vi "VersionStrings.GetProjectPaths.vi"(1 "Version Build Info":T1={"VeriStand Version"="2013 SP1", "TestStand Version"="2013", "New VS Assembly Version"="2013.0.0.0", "New TS Assembly Version"="5.1.0.226", "VeriStand Steps Version String"="14.0.5.0", "Project Paths"={"MiscHelperVIs Project Path"="", "RTSequenceVIs Project Path"="", "Set Channels Project Path"="", "TS VS Logger Project Path"="", "VeriStand.exe Install Path"="", "NI_VeristandTypes.ini File Path"="", "Workspace Path"="", "VeristandSteps.csproj File Path"="", "Silent Veristand Project Path"=""}, "New TS Interop Assembly Version"="1.2.3.4", "New TS Utility Assembly Version"="5.6.7.8", "New VS Assembly Version (GAC)"="4.0.2016.0.9.9", "dotNET .config File Paths"={"MiscHelperVIs Project .config File Path"=path "C:/Users/Public/Documents/Git-Source/VeriStand-Custom-Steps-For-TestStand/Source/LabVIEW Code/Misc/MiscHelperVIs.lvproj.config", "RT Sequence VIs Project .config File Path"=path "C:/Users/Public/Documents/Git-Source/VeriStand-Custom-Steps-For-TestStand/Source/LabVIEW Code/RT Sequence/RTSequenceVIs.lvproj.config", "Set Channels Project .config File Path"=path "C:/Users/Public/Documents/Git-Source/VeriStand-Custom-Steps-For-TestStand/Source/LabVIEW Code/Set Channels/Set Channels.lvproj.config", "TS VS Logger Project .config File Path"=path "C:/Users/Public/Documents/Git-Source/VeriStand-Custom-Steps-For-TestStand/Source/LabVIEW Code/TS VS Logger/TS VS Logger.lvproj.config", "Silent Veristand Project .config File Path"=path "C:/Users/Public/Documents/Git-Source/VeriStand-Custom-Steps-For-TestStand/Source/LabVIEW Code/VeriStand Silent Start/SilentVS.lvproj.config"}}) -> (0 "Version Build Info out":T1={"VeriStand Version"="2013 SP1", "TestStand Version"="2013", "New VS Assembly Version"="2013.0.0.0", "New TS Assembly Version"="5.1.0.226", "VeriStand Steps Version String"="14.0.5.0", "Project Paths"={"MiscHelperVIs Project Path"="", "RTSequenceVIs Project Path"="", "Set Channels Project Path"="", "TS VS Logger Project Path"="", "VeriStand.exe Install Path"="", "NI_VeristandTypes.ini File Path"="", "Workspace Path"="", "VeristandSteps.csproj File Path"="", "Silent Veristand Project Path"=""}, "New TS Interop Assembly Version"="1.2.3.4", "New TS Utility Assembly Version"="5.6.7.8", "New VS Assembly Version (GAC)"="4.0.2016.0.9.9", "dotNET .config File Paths"={"MiscHelperVIs Project .config File Path"=path "C:/Users/Public/Documents/Git-Source/VeriStand-Custom-Steps-For-TestStand/Source/LabVIEW Code/Misc/MiscHelperVIs.lvproj.config", "RT Sequence VIs Project .config File Path"=path "C:/Users/Public/Documents/Git-Source/VeriStand-Custom-Steps-For-TestStand/Source/LabVIEW Code/RT Sequence/RTSequenceVIs.lvproj.config", "Set Channels Project .config File Path"=path "C:/Users/Public/Documents/Git-Source/VeriStand-Custom-Steps-For-TestStand/Source/LabVIEW Code/Set Channels/Set Channels.lvproj.config", "TS VS Logger Project .config File Path"=path "C:/Users/Public/Documents/Git-Source/VeriStand-Custom-Steps-For-TestStand/Source/LabVIEW Code/TS VS Logger/TS VS Logger.lvproj.config", "Silent Veristand Project .config File Path"=path "C:/Users/Public/Documents/Git-Source/VeriStand-Custom-Steps-For-TestStand/Source/LabVIEW Code/VeriStand Silent Start/SilentVS.lvproj.config"}})   [LabVIEW 2014, in "VeriStand Steps Version Mutation.lvlib"]
uses:
  VeriStand Steps Version Mutation.lvlib
  Types/Version Build Information.ctl
  Types/Project Paths Cluster.ctl
  Types/dotNET Config File Paths Cluster.ctl
  Types/Constants.vi
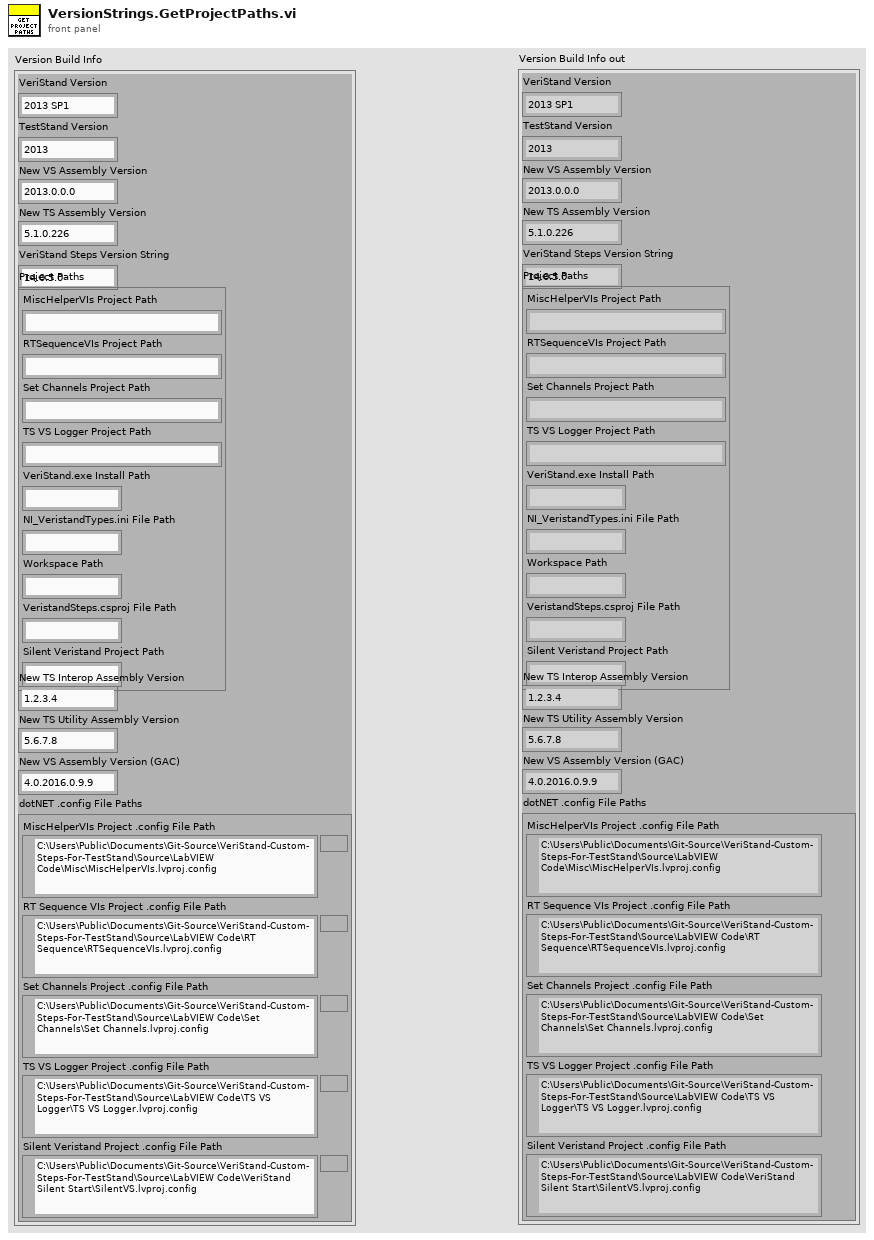
[diagram p1: front panel]
types:
  T1 = typedef "VeriStand Steps Version Mutation.lvlib/Version Build Information.ctl" = cluster{"VeriStand Version":string, "TestStand Version":string, "New VS Assembly Version":string, "New TS Assembly Version":string, "VeriStand Steps Version String":string, "Project Paths":T2, "New TS Interop Assembly Version":string, "New TS Utility Assembly Version":string, "New VS Assembly Version (GAC)":string, "dotNET .config File Paths":T3}
  T2 = typedef "VeriStand Steps Version Mutation.lvlib/Project Paths Cluster.ctl" = cluster{"MiscHelperVIs Project Path":string, "RTSequenceVIs Project Path":string, "Set Channels Project Path":string, "TS VS Logger Project Path":string, "VeriStand.exe Install Path":string, "NI_VeristandTypes.ini File Path":string, "Workspace Path":string, "VeristandSteps.csproj File Path":string, "Silent Veristand Project Path":string}
  T3 = typedef "VeriStand Steps Version Mutation.lvlib/dotNET Config File Paths Cluster.ctl" = cluster{"MiscHelperVIs Project .config File Path":path, "RT Sequence VIs Project .config File Path":path, "Set Channels Project .config File Path":path, "TS VS Logger Project .config File Path":path, "Silent Veristand Project .config File Path":path}
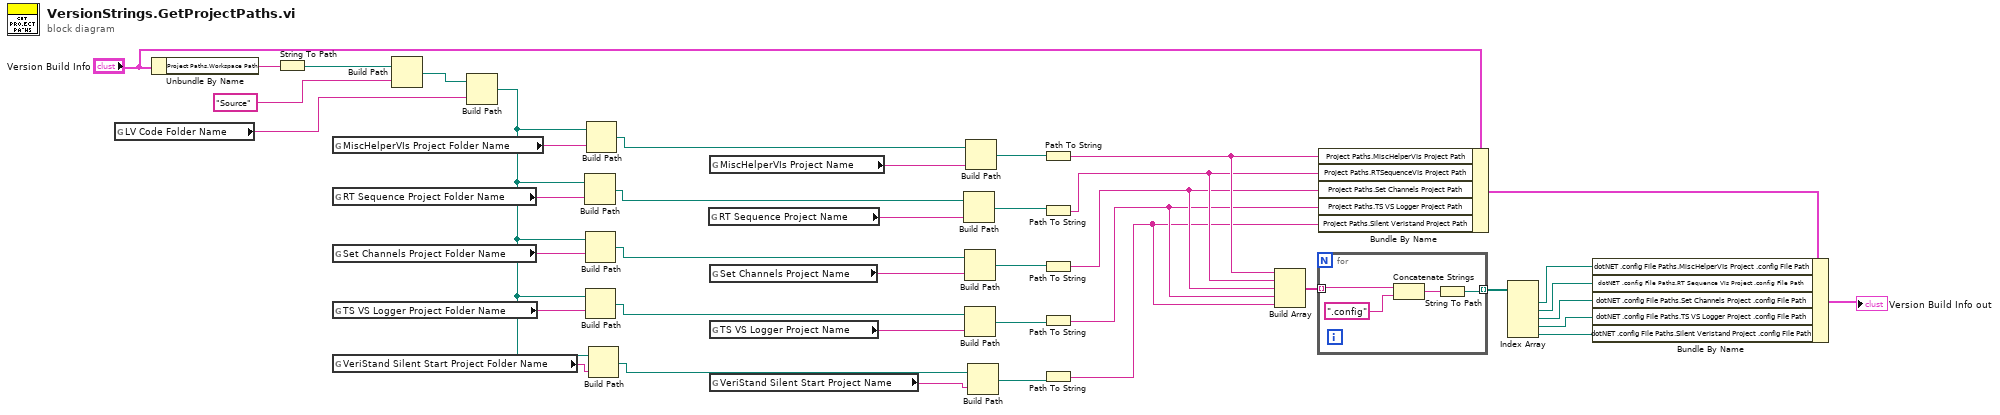
[diagram p0: block diagram]
diagram:
  n1 = global read "Constants.vi" "LV Code Folder Name"() -> (w38:string)
  n2 = Unbundle By Name("Version Build Info") -> ("Project Paths.Workspace Path"=w41:string)
  n3 = String To Path(string=w41) -> (path=w40:path)
  n4 = global read "Constants.vi" "MiscHelperVIs Project Folder Name"() -> (w37:string)
  n5 = global read "Constants.vi" "RT Sequence Project Folder Name"() -> (w35:string)
  n6 = global read "Constants.vi" "Set Channels Project Folder Name"() -> (w34:string)
  n7 = global read "Constants.vi" "TS VS Logger Project Folder Name"() -> (w33:string)
  n8 = global read "Constants.vi" "VeriStand Silent Start Project Folder Name"() -> (w31:string)
  n9 = Build Path(base path=w40, name or relative path="Source") -> (appended path=w36:path)
  n10 = Build Path(base path=w36, name or relative path=w38) -> (appended path=w32:path)
  n11 = Build Path(base path=w32, name or relative path=w35) -> (appended path=w29:path)
  n12 = Build Path(base path=w32, name or relative path=w34) -> (appended path=w28:path)
  n13 = Build Path(base path=w32, name or relative path=w33) -> (appended path=w27:path)
  n14 = Build Path(base path=w32, name or relative path=w37) -> (appended path=w30:path)
  n15 = Build Path(base path=w32, name or relative path=w31) -> (appended path=w26:path)
  n16 = global read "Constants.vi" "RT Sequence Project Name"() -> (w24:string)
  n17 = global read "Constants.vi" "MiscHelperVIs Project Name"() -> (w25:string)
  n18 = global read "Constants.vi" "Set Channels Project Name"() -> (w23:string)
  n19 = global read "Constants.vi" "TS VS Logger Project Name"() -> (w22:string)
  n20 = global read "Constants.vi" "VeriStand Silent Start Project Name"() -> (w21:string)
  n21 = Build Path(base path=w29, name or relative path=w24) -> (appended path=w18:path)
  n22 = Build Path(base path=w28, name or relative path=w23) -> (appended path=w17:path)
  n23 = Build Path(base path=w27, name or relative path=w22) -> (appended path=w16:path)
  n24 = Build Path(base path=w30, name or relative path=w25) -> (appended path=w19:path)
  n25 = Build Path(base path=w26, name or relative path=w21) -> (appended path=w15:path)
  n26 = Path To String(path=w19) -> (string=w14:string)
  n27 = Path To String(path=w18) -> (string=w13:string)
  n28 = Path To String(path=w17) -> (string=w12:string)
  n29 = Path To String(path=w16) -> (string=w11:string)
  n30 = Path To String(path=w15) -> (string=w10:string)
  n31 = Build Array(w14, w13, w12, w11, w10) -> (w9:string[])
  n32 = for {
    tunnel: w9 -> [w45] mode=indexing
    tunnel: [w42] -> w7 mode=indexing
    n33 = Concatenate Strings(w45, ".config" ("string")) -> (w43:string)
    n34 = String To Path(string=w43) -> (path=w42:path)
  }
  n35 = Bundle By Name(cluster="Version Build Info", "Project Paths.MiscHelperVIs Project Path"=w14, "Project Paths.RTSequenceVIs Project Path"=w13, "Project Paths.Set Channels Project Path"=w12, "Project Paths.TS VS Logger Project Path"=w11, "Project Paths.Silent Veristand Project Path"=w10) -> (w8:T1)
  n36 = Index Array(array=w7) -> (element #1=w6:path, element #2=w5:path, element #3=w4:path, element #4=w3:path, element #5=w2:path)  [unwired: 5 in]
  n37 = Bundle By Name(cluster=w8, "dotNET .config File Paths.MiscHelperVIs Project .config File Path"=w6, "dotNET .config File Paths.RT Sequence VIs Project .config File Path"=w5, "dotNET .config File Paths.Set Channels Project .config File Path"=w4, "dotNET .config File Paths.TS VS Logger Project .config File Path"=w3, "dotNET .config File Paths.Silent Veristand Project .config File Path"=w2) -> (→"Version Build Info out":T1)
